vi "Pick and Place Tool.vi"   [LabVIEW 2016]
uses:
  Drivers/Aerotech A3200/Aerotech VIs.lvlib
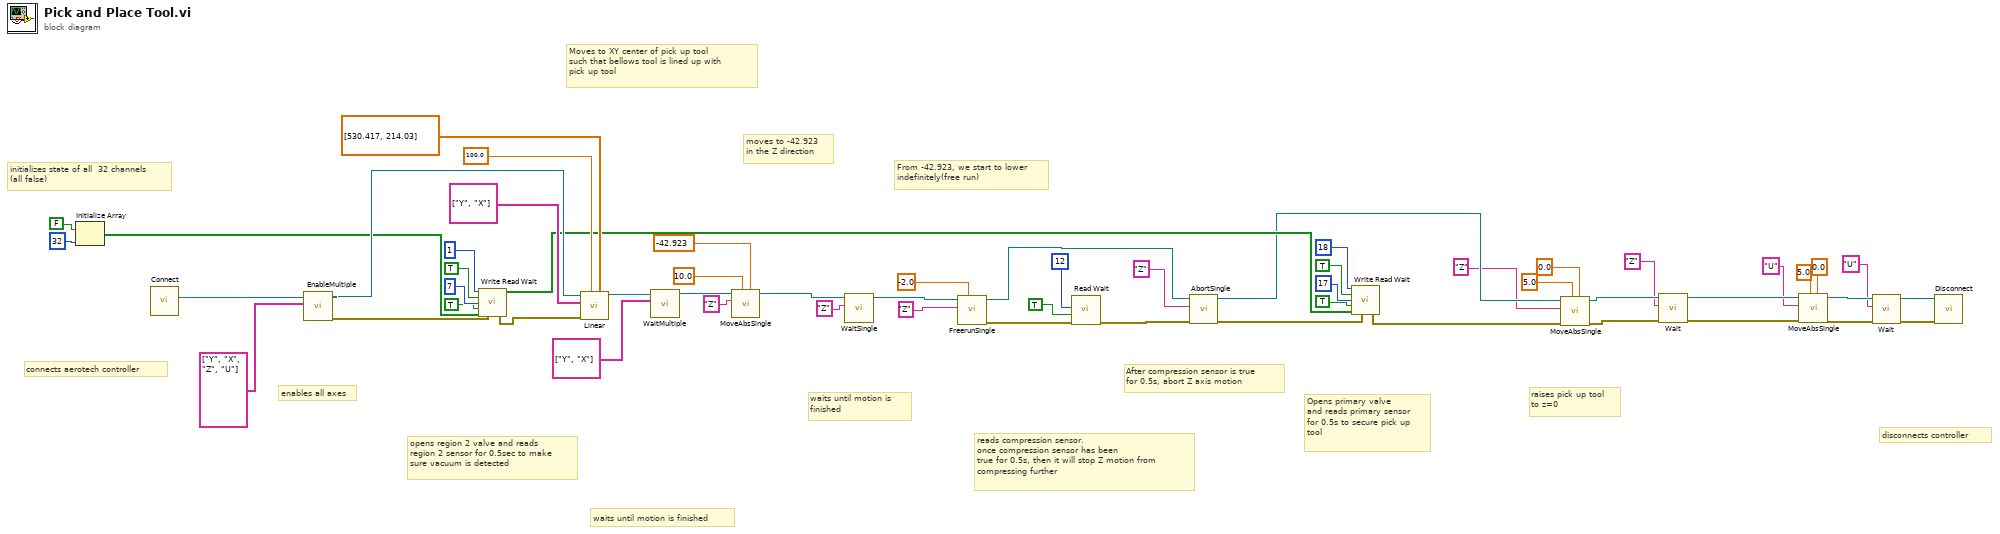
[diagram p0: block diagram]
diagram:
  # "disconnects controller"
  # "raises pick up tool\nto z=0"
  # "Opens primary valve \nand reads primary sensor\nfor 0.5s to secure pick up\ntool"
  # "After compression sensor is true\nfor 0.5s, abort Z axis motion"
  # "reads compression sensor.\nonce compression sensor has been \ntrue for 0.5s, then it will stop Z motion from \ncompressing further"
  # "From -42.923, we start to lower\nindefinitely(free run)"
  # "waits until motion is\nfinished"
  # "moves to -42.923 \nin the Z direction"
  # "waits until motion is finished"
  # "Moves to XY center of pick up tool\nsuch that bellows tool is lined up with \npick up tool"
  # "opens region 2 valve and reads\nregion 2 sensor for 0.5sec to make\nsure vacuum is detected"
  # "enables all axes"
  # "connects aerotech controller"
  # "initializes state of all  32 channels\n(all false)"
  n1 = Initialize Array(FALSE, 32) -> (w31:bool[])
  n2 = call "Connect.vi"() -> ("controller"=w56:refnum<k24>)  [unwired: 10 in, 1 out]
  n3 = call "EnableMultiple.vi"("axis names"=string[] ["Y", "X", "Z", "U"], "controller in"=w56) -> ("error out"=w39:errorcluster, "controller out"=w54:refnum<k24>)  [unwired: 8 in]
  n4 = call "Write Read Wait.vi"("Valve Channel"=1, "Open/ Close Valve"=TRUE, "Sensor Channel"=7, "Desired Sensor Value"=TRUE, "Initial State"=w31, "error in (no error)"=w39) -> ("FinalState"=w20:bool[], "error out"=w38:errorcluster)  [unwired: 8 in]
  n5 = call "Linear.vi"("distances"=dbl[] [530.417, 214.03], "speed"=100.0, "error in (no error)"=w38, "axis names"=string[] ["Y", "X"], "controller in"=w54) -> ("controller out"=w49:refnum<k24>)  [unwired: 5 in, 1 out]
  n6 = call "WaitMultiple.vi"("axis names"=string[] ["Y", "X"], "controller in"=w49) -> ("controller out"=w48:refnum<k24>)  [unwired: 7 in, 2 out]
  n7 = call "MoveAbsSingle.vi"("position"=-42.923, "speed"=10.0, "axis name"="Z", "controller in"=w48) -> ("controller out"=w44:refnum<k24>)  [unwired: 6 in, 1 out]
  n8 = call "WaitSingle.vi"("axis name"="Z", "controller in"=w44) -> ("controller out"=w42:refnum<k24>)  [unwired: 7 in, 2 out]
  n9 = call "FreerunSingle.vi"("speed"=-2.0, "axis name"="Z", "controller in"=w42) -> ("error out"=w30:errorcluster, "controller out"=w14:refnum<k24>)  [unwired: 7 in]
  n10 = call "Read Wait.vi"("Sensor Channel"=12, "Desired Value"=TRUE, "error in (no error)"=w30) -> ("error out"=w27:errorcluster)  [unwired: 7 in]
  n11 = call "AbortSingle.vi"("error in (no error)"=w27, "axis name? (all)"="Z", "controller in"=w14) -> ("error out"=w25:errorcluster, "controller out"=w18:refnum<k24>)  [unwired: 7 in]
  n12 = call "Write Read Wait.vi"("Valve Channel"=18, "Open/ Close Valve"=TRUE, "Sensor Channel"=17, "Desired Sensor Value"=TRUE, "Initial State"=w20, "error in (no error)"=w25) -> ("error out"=w19:errorcluster)  [unwired: 8 in, 1 out]
  n13 = call "MoveAbsSingle.vi"("position"=0.0, "speed"=5.0, "error in (no error)"=w19, "axis name"="Z", "controller in"=w18) -> ("error out"=w10:errorcluster, "controller out"=w11:refnum<k24>)  [unwired: 5 in]
  n14 = call-poly "Wait.vi"("error in (no error)"=w10, "axis name"="Z", "controller in"=w11) -> ("error out"=w13:errorcluster, "controller out"=w12:refnum<k24>)  [unwired: 6 in, 1 out]
  n15 = call "MoveAbsSingle.vi"("position"=0.0, "speed"=5.0, "error in (no error)"=w13, "axis name"="U", "controller in"=w12) -> ("error out"=w9:errorcluster, "controller out"=w7:refnum<k24>)  [unwired: 5 in]
  n16 = call-poly "Wait.vi"("error in (no error)"=w9, "axis name"="U", "controller in"=w7) -> ("error out"=w8:errorcluster, "controller out"=w6:refnum<k24>)  [unwired: 6 in, 1 out]
  n17 = call "Disconnect.vi"("error in (no error)"=w8, "controller"=w6) -> ()  [unwired: 9 in, 1 out]
